vi "Compute Turns(2pt).vi"(9 "Long Offset":dbl, 11 "Short Offset":dbl) -> (3 "Turns Clockwise":dbl format="%.3f")   [LabVIEW 2019]
uses:
  <vilib>/Analysis/6fits.llb/Curve Fitting Criteria.ctl
  Analysis/Global Tube Measurement.vi
  <vilib>/Analysis/NI_AALPro.lvlib
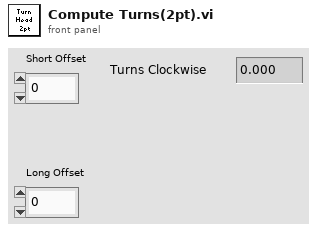
[diagram p1: front panel]
types:
  T1 = typedef "NI_AALPro.lvlib/Curve Fitting Criteria.ctl" = u16
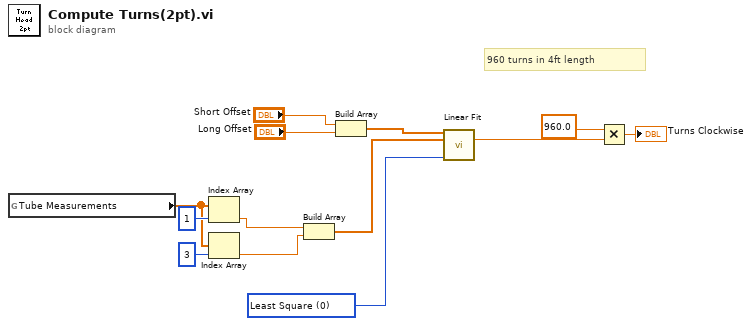
[diagram p0: block diagram]
diagram:
  w7 = T1 0 items=["Least Square", "Least Absolute Residual", "Bisquare"] ("method")
  # "960 turns in 4ft length"
  n1 = global read "Global Tube Measurement.vi" "Tube Measurements"() -> (w4:dbl[])
  n2 = Index Array(array=w4, index=1) -> (element=w3:dbl)
  n3 = Index Array(array=w4, index=3) -> (element=w2:dbl)
  n4 = Build Array(w3, w2) -> (w1:dbl[])
  n5 = Build Array("Short Offset", "Long Offset") -> (w10:dbl[])
  n6 = call <vilib>:"Linear Fit.vi"("Y"=w10, "X"=w1, "method"=w7) -> ("slope"=w12:dbl)  [unwired: 8 in, 4 out]
  n7 = Multiply(x=960.0 ("Offset 3"), y=w12) -> (x*y=→"Turns Clockwise":dbl)
